vi "Get Terminals.vi"(8 "error in (no error)":errorcluster, 10 "to object reference":i32, 11 "Data Cluster in":T1) -> (0 "error out":errorcluster, 2 "Terms[]":refnum<vi>[](array[refnum]), 3 "Data Cluster out":T1)   [LabVIEW 2025, in "Scripting Server.lvlib"]
uses:
  Scripting Server.lvlib
  Module Data--cluster.ctl
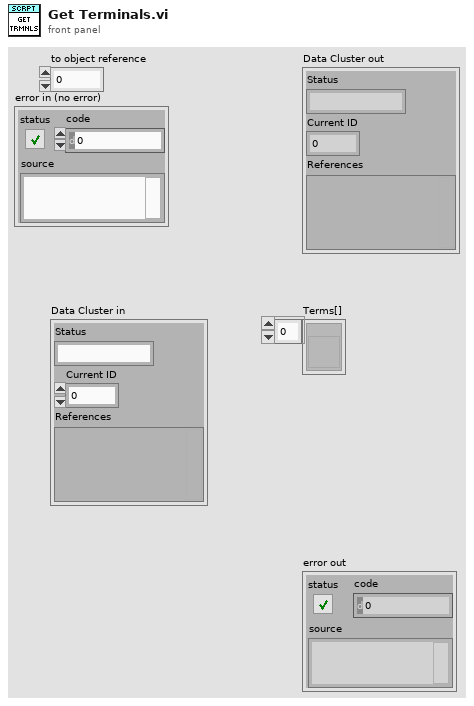
[diagram p1: front panel]
types:
  T1 = typedef "Scripting Server.lvlib/Module Data--cluster.ctl" = cluster{"Status":string, "Current ID":i32, "References":variant}
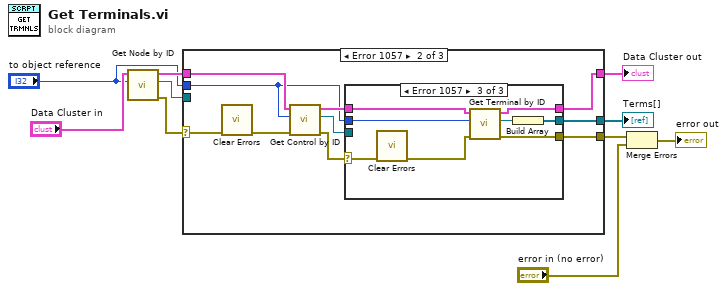
[diagram p0: block diagram]
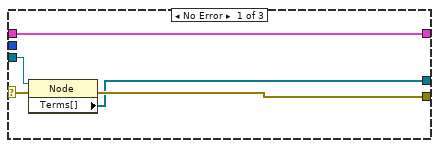
[diagram p2: hidden frame]
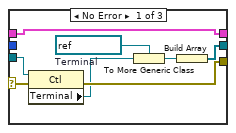
[diagram p3: hidden frame]
diagram:
  n1 = call "Get Node by ID.vi"("ID"="to object reference", "Data Cluster in"="Data Cluster in") -> ("error out"=w6:errorcluster, "specific class reference"=w9:refnum<vi>, "Data Cluster out"=w5:T1)  [unwired: 7 in]
  n2 = case shown="Error 1057" w6 {
    selector: w6 -> [w12 w25 w45]
    tunnel: [w15 w23 w45] -> w10
    tunnel: w9 -> [w14 _ _]
    tunnel: [w13 w21 _] -> w7
    tunnel: w5 -> [w11 w24 w44]
    tunnel: [w11 w17 w44] -> w4
    tunnel: "to object reference" -> [_ w16 _]
    frame No Error {
      n3 = property class="Node"(reference=w14, error in=w12) -> (error out=w15:errorcluster, "Terms[]"=w13:refnum<vi>[])  [unwired: 1 out]
    }
    frame Error {
      n4 = call <vilib>:"Clear Errors.vi"("error in (no error)"=w25) -> ("error out"=w20:errorcluster)  [unwired: 5 in, 1 out]
      n5 = call "Get Control by ID.vi"("error in (no error)"=w20, "ID"=w16, "Data Cluster in"=w24) -> ("error out"=w19:errorcluster, "specific class reference"=w22:refnum<vi>, "Data Cluster out"=w18:T1)  [unwired: 6 in]
      n6 = case shown="Error 1057" w19 {
        selector: w19 -> [w29 w35 w43]
        tunnel: [w33 w35 w41] -> w23
        tunnel: w22 -> [w32 _ _]
        tunnel: [w30 _ w36] -> w21
        tunnel: w18 -> [w28 w34 w40]
        tunnel: [w28 w34 w39] -> w17
        tunnel: w16 -> [_ _ w38]
        frame No Error {
          w26 = refnum<vi> refnum  # Terminal
          n7 = property class="Ctl"(reference=w32, error in=w29) -> (error out=w33:errorcluster, "Terminal"=w31:refnum<vi>)  [unwired: 1 out]
          n8 = To More Generic Class(target class=w26, reference=w31) -> (generic class reference=w27:refnum<vi>)
          n9 = Build Array(w27) -> (w30:refnum<vi>[])
        }
        frame Default {
        }
        frame Error {
          n10 = call <vilib>:"Clear Errors.vi"("error in (no error)"=w43) -> ("error out"=w42:errorcluster)  [unwired: 5 in, 1 out]
          n11 = call "Get Terminal by ID.vi"("error in (no error)"=w42, "ID"=w38, "Data Cluster in"=w40) -> ("error out"=w41:errorcluster, "specific class reference"=w37:refnum<vi>, "Data Cluster out"=w39:T1)  [unwired: 6 in]
          n12 = Build Array(w37) -> (w36:refnum<vi>[])
        }
      }
    }
    frame Default {
    }
  }
  "Data Cluster out" <- w4
  "Terms[]" <- w7
  n13 = Merge Errors(w10, "error in (no error)") -> (→"error out":errorcluster)
